vi "Set Paths.vi"(7 "Measurement specfic paths":T1=enum."Harmonics", 8 "error in (no error)":errorcluster, 11 "Path Switch in":refnum<class "Path Switch.lvclass">) -> (0 "error out":errorcluster, 3 "Path Switch out":refnum<class "Path Switch.lvclass">)   [LabVIEW 2020, in "Path Switch.lvclass"]
uses:
  Path Switch.lvclass
  Path Control/Measurements Specific Paths.ctl
  Path Control/PathControl.lvclass
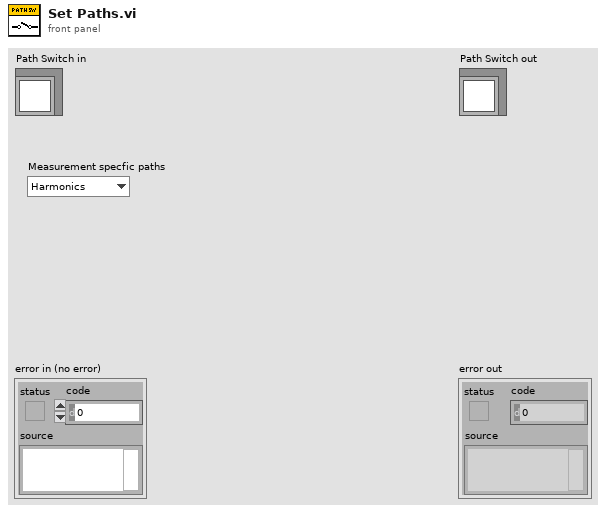
[diagram p1: front panel]
types:
  T1 = typedef "PathControl.lvclass/Measurements Specific Paths.ctl" = enum16{"No calibration", "Harmonics", "IMD", "S Parameter", "AM-AM", "MCCW-ACLR", "DC", "LCR", "Power Meter GUI", "RF Power"}
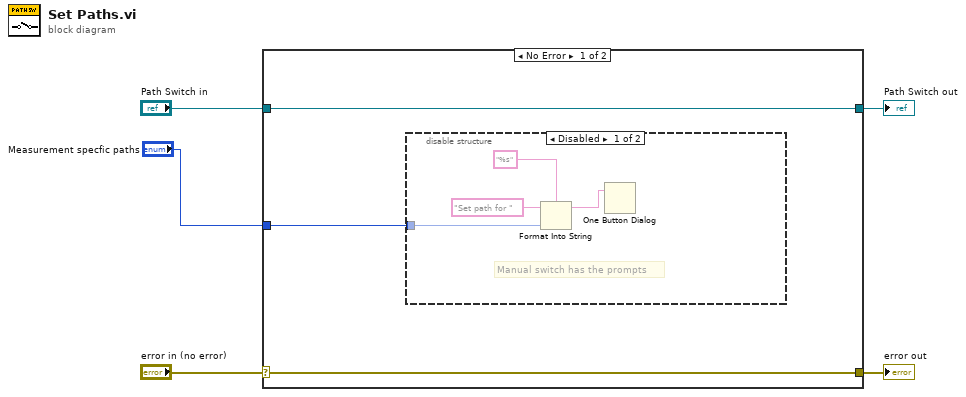
[diagram p0: block diagram]
diagram:
  n1 = case shown="No Error" "error in (no error)" {
    selector: "error in (no error)" -> [w7 w14]
    tunnel: [w7 w14] -> w4
    tunnel: [w8 w13] -> w2
    tunnel: "Path Switch in" -> [w8 w13]
    tunnel: "Measurement specfic paths" -> [w6 _]
    frame No Error {
      n2 = disable-structure shown="Disabled" {
        disable-tunnel: w6 -> [w9 _]
        frame Disabled {
          # "Manual switch has the prompts"
          n3 = Format Into String(format string="%s", initial string="Set path for ", w9) -> (resulting string=w10:string)  [unwired: 1 in, 1 out]
          n4 = One Button Dialog(message=w10) -> ()  [unwired: 1 in, 1 out]
        }
        frame Enabled {
        }
      }
    }
    frame Error {
    }
  }
  "error out" <- w4
  "Path Switch out" <- w2
